vi "Get DataRateLevel.vi"(6 "timeout (ms)":i32=-1, 8 "error in (no error)":errorcluster, 10 "channel_name":string, 11 "FlexLogger_gRPC in":refnum<class "FlexLogger_gRPC.lvclass">) -> (0 "error out":errorcluster, 2 "Data Rate Level":T1, 3 "FlexLogger_gRPC out":refnum<class "FlexLogger_gRPC.lvclass">)   [LabVIEW 2020, in "FlexLogger_gRPC.lvlib" / "FlexLogger_gRPC.lvclass"]
doc: "Gets the data rate level of the subsystem that owns a channel."
uses:
  FlexLogger_gRPC.lvclass
  Controls/Flexlogger Data Rate Level Enum.ctl
  FlexLogger_client/RPC Messages/flexlogger_GetDataRateLevelRequest.ctl
  FlexLogger_client/RPC Messages/flexlogger_ElementIdentifier.ctl
  FlexLogger_gRPC.lvclass/FlexLogger_gRPC.ctl
  FlexLogger_client/FlexLogger_client.lvlib
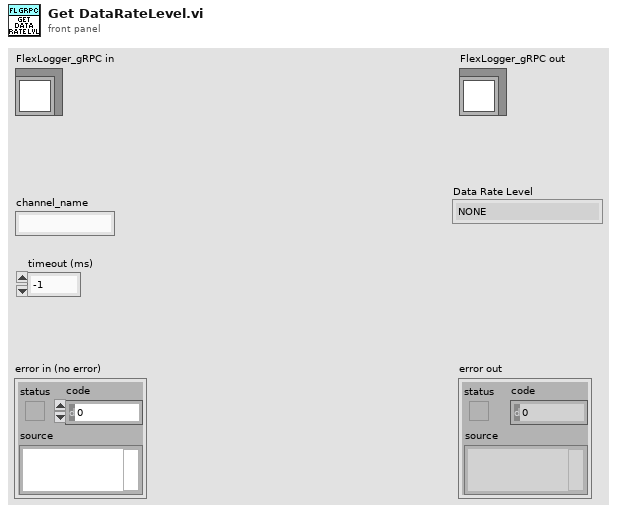
[diagram p1: front panel]
types:
  T1 = typedef "FlexLogger_gRPC.lvlib/FlexLogger_gRPC.lvclass/Flexlogger Data Rate Level Enum.ctl" = enum16{"NONE", "SLOW", "MEDIUM", "FAST", "COUNTER", "DIGITAL", "ON DEMAND"}
  T2 = typedef "FlexLogger_client.lvlib/flexlogger_GetDataRateLevelRequest.ctl" = cluster{"document_identifier":T3, "channel_name":string}
  T3 = typedef "FlexLogger_client.lvlib/flexlogger_ElementIdentifier.ctl" = cluster{"project_id":string, "file_name":string, "element_id":string, "subpart_id":string}
  T4 = typedef "grpc-lvsupport-release.lvlib/grpcId.ctl" = u64
  T5 = typedef "FlexLogger_client.lvlib/flexlogger_GetDataRateLevelResponse.ctl" = cluster{"data_rate_level":i32}
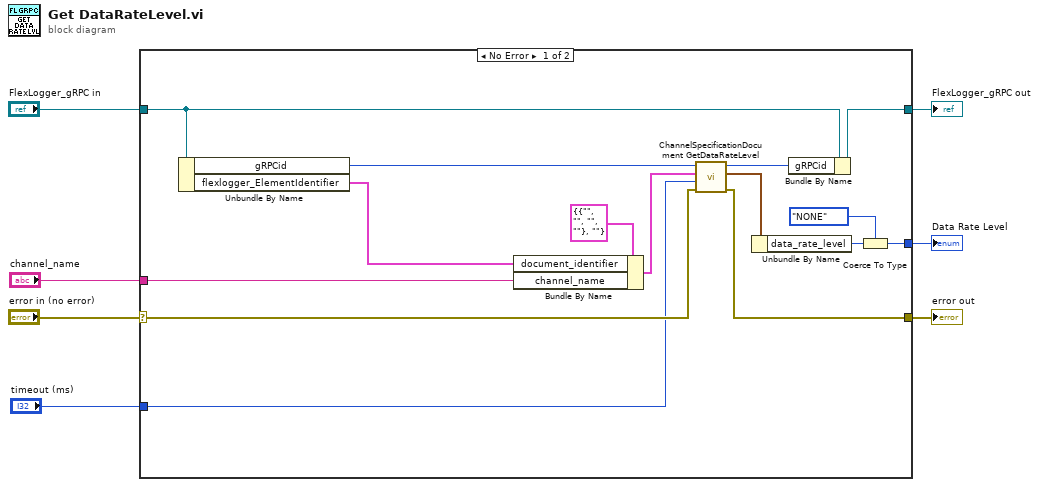
[diagram p0: block diagram]
diagram:
  n1 = case shown="No Error" "error in (no error)" {
    selector: "error in (no error)" -> [w21 w23]
    tunnel: "FlexLogger_gRPC in" -> [w20 w24]
    tunnel: [w19 w24] -> w7
    tunnel: [w17 w23] -> w5
    tunnel: [w15 _] -> w3
    tunnel: "channel_name" -> [w12 _]
    tunnel: "timeout (ms)" -> [w13 _]
    frame No Error {
      n2 = Unbundle By Name(w20) -> ("gRPCid"=w22:T4, "flexlogger_ElementIdentifier"=w11:T3)
      n3 = Bundle By Name(cluster=T2 {"document_identifier"={"project_id"="", "file_name"="", "element_id"="", "subpart_id"=""}, "channel_name"=""} ("Request Data"), "document_identifier"=w11, "channel_name"=w12) -> (w8:T2)
      n4 = call "ChannelSpecificationDocument GetDataRateLevel.vi"("error in"=w21, "timeout (ms)"=w13, "Request Data"=w8, "gRPC ID"=w22) -> ("error out"=w17:errorcluster, "Response Data"=w10:T5, "gRPC ID out"=w18:T4)  [unwired: 5 in]
      n5 = Unbundle By Name(w10) -> ("data_rate_level"=w16:i32)
      n6 = Bundle By Name(cluster=w20, "gRPCid"=w18) -> (w19:refnum<class "FlexLogger_gRPC.lvclass">)
      n7 = Coerce To Type(0:w16, 1:Flexlogger_Data_Rate_Level_Enum."NONE" ("Data Rate Level")) -> (2:w15:T1)
    }
    frame Error {
    }
  }
  "error out" <- w5
  "FlexLogger_gRPC out" <- w7
  "Data Rate Level" <- w3
